vi "GetCellHeight.vi"(4 "error in (no error)":errorcluster, 6 "Container State":T2, 7 "Display State In":T1={"Items"=[{"Tag"="1", "Name"="1", "Symbol"=0, "Checked"=FALSE, "ParentTag"="t"}], "CellHeight"=0}) -> (0 "error out":errorcluster, 2 "Value":i32, 3 "Display State Out":T1={"Items"=[{"Tag"="1", "Name"="1", "Symbol"=0, "Checked"=FALSE, "ParentTag"="t"}], "CellHeight"=0})   [LabVIEW 2020, in "XSubMenu.xctl"]
uses:
  XSubMenu.xctl
  <vilib>/_xctls/Container State.ctl
  XSubMenu-State.ctl
  <vilib>/_xctls/XControlSupport.lvlib
panel:
  # "Replace the Value Indicator below with an Indicator of desired type.\nDo not remove this Indicator or the others from the connector pane. \nDo not change the connector pane pattern.\nThe Value Indicator should always be the second terminal from top on the output side in the connector pane."
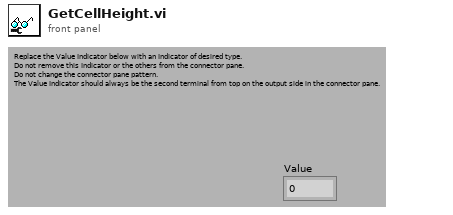
[diagram p1: front panel]
types:
  T1 = typedef "XSubMenu.xctl/XSubMenu-State.ctl" = cluster{"Items":cluster{"Tag":string, "Name":string, "Symbol":i32, "Checked":bool, "ParentTag":string}[], "CellHeight":i32}
  T2 = typedef "XControlSupport.lvlib/Container State.ctl" = cluster{"Indicator?":bool, "Run Mode?":bool, " Refnum":refnum<vi>}
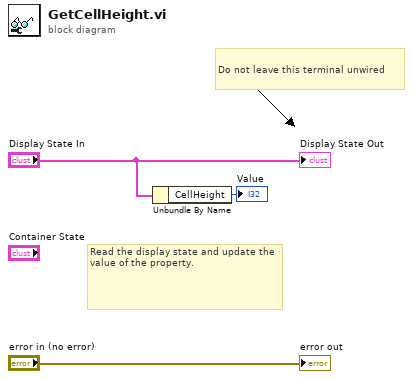
[diagram p0: block diagram]
diagram:
  # "Do not leave this terminal unwired"
  # "Read the display state and update the value of the property."
  n1 = Unbundle By Name("Display State In") -> ("CellHeight"=→"Value":i32)
  "error out" <- "error in (no error)"
  "Display State Out" <- "Display State In"
